vi "Module - RH_RABAR.vi"() -> ()   [LabVIEW 2019]
uses:
  Control/State - eFGV.ctl
panel:
  out "Site Name":string="RH JONATHAN (13.65 kWp)"
  out "STP-03-STATUS":bool
  out "STP-03-B-IDC":dbl caption="B.Idc" format="%.1f A"
  out "STP-03-B-VDC":dbl caption="B.Vdc" format="%.0f V"
  out "STP-03-A-IDC":dbl caption="A.Idc" format="%.1f A"
  out "STP-03-A-VDC":dbl caption="A.Vdc" format="%.0f V"
  out "STP-03-PAC":dbl caption="Pac" format="%#_g W"
  out "BANK-02-TEMP":dbl caption="T_bat" format="%#_g C"
  out "BANK-02-IDC":dbl caption="I_bat" format="%.2f A"
  out "BANK-02-VDC":dbl caption="V_bat" format="%.1f V"
  out "BANK-02-SOC":dbl caption="SOC" format="%#_g %"
  out "PM-01-STATUS":bool
  out "PM-01-FREQ":dbl caption="Freq" format="%.0f Hz"
  out "PM-01-IAC":dbl caption="Iac" format="%.0f A"
  out "PM-01-VAC":dbl caption="Vac" format="%.0f V"
  out "PM-01-PAC":dbl caption="Pac" format="%.0f W"
  out "SI-M-01-STATUS":bool
  out "SI-M-01-FREQ":dbl caption="FREQ" format="%.0f Hz"
  out "SI-M-01-L3":dbl caption="L3" format="%.0f V"
  out "SI-M-01-L2":dbl caption="L2" format="%.0f V"
  out "SI-M-01-L1":dbl caption="L1" format="%.0f V"
  out "SI-M-01-PAC":dbl caption="Pac" format="%.0f W"
  out "BANK-01-TEMP":dbl caption="T_bat" format="%#_g C"
  out "BANK-01-IDC":dbl caption="I_bat" format="%.2f A"
  out "BANK-01-VDC":dbl caption="V_bat" format="%.1f V"
  out "BANK-01-SOC":dbl caption="SOC" format="%#_g %"
  out "STP-02-STATUS":bool
  out "STP-02-B-IDC":dbl caption="B.Idc" format="%.1f A"
  out "STP-02-B-VDC":dbl caption="B.Vdc" format="%.0f V"
  out "STP-02-A-IDC":dbl caption="A.Idc" format="%.1f A"
  out "STP-02-A-VDC":dbl caption="A.Vdc" format="%.0f V"
  out "STP-02-PAC":dbl caption="Pac" format="%#_g W"
  out "STP-01-STATUS":bool
  out "STP-01-B-IDC":dbl caption="B.Idc" format="%.1f A"
  out "STP-01-B-VDC":dbl caption="B.Vdc" format="%.0f V"
  out "STP-01-A-IDC":dbl caption="A.Idc" format="%.1f A"
  out "STP-01-A-VDC":dbl caption="A.Vdc" format="%.0f V"
  out "STP-01-PAC":dbl caption="Pac" format="%.0f W"
  # "RH RABAR (17.29 kWp)"
  # "BANK-1"
  # "BANK-2"
  # "STP-01"
  # "STP-02"
  # "SI-M-01"
  # "STP-03"
  # "PM-01"
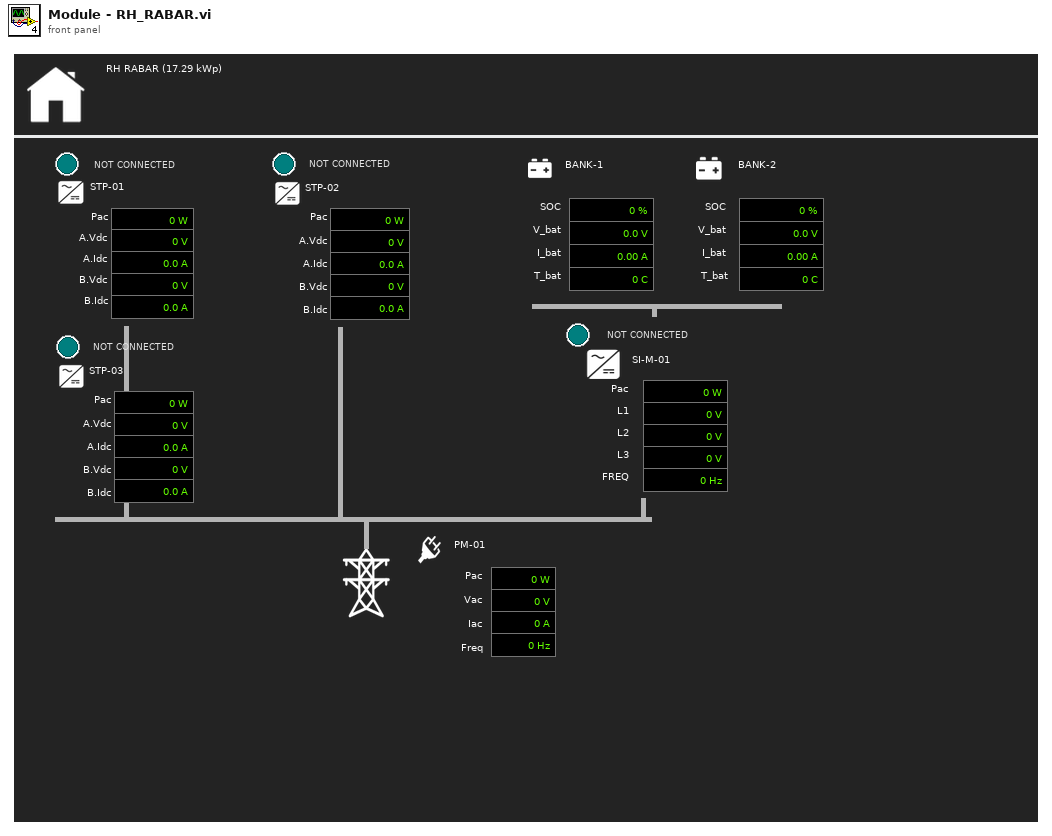
[diagram p1: front panel]
types:
  T1 = typedef "State - eFGV.ctl" = enum16{"Init", "Read", "Write", "Close"}
  T2 = typedef "Device Name.ctl" = enum16{"SB-01", "SB-02", "SB-03", "SB-04", "STP-01", "STP-02", "STP-03", "STP-04", "BANK-01", "BANK-02", "BANK-03", "BANK-04", "SI-M-01", "SI-M-02", "SI-M-03", "SI-M-04", "PM-01", "PM-02", "PM-03", "PM-04"}
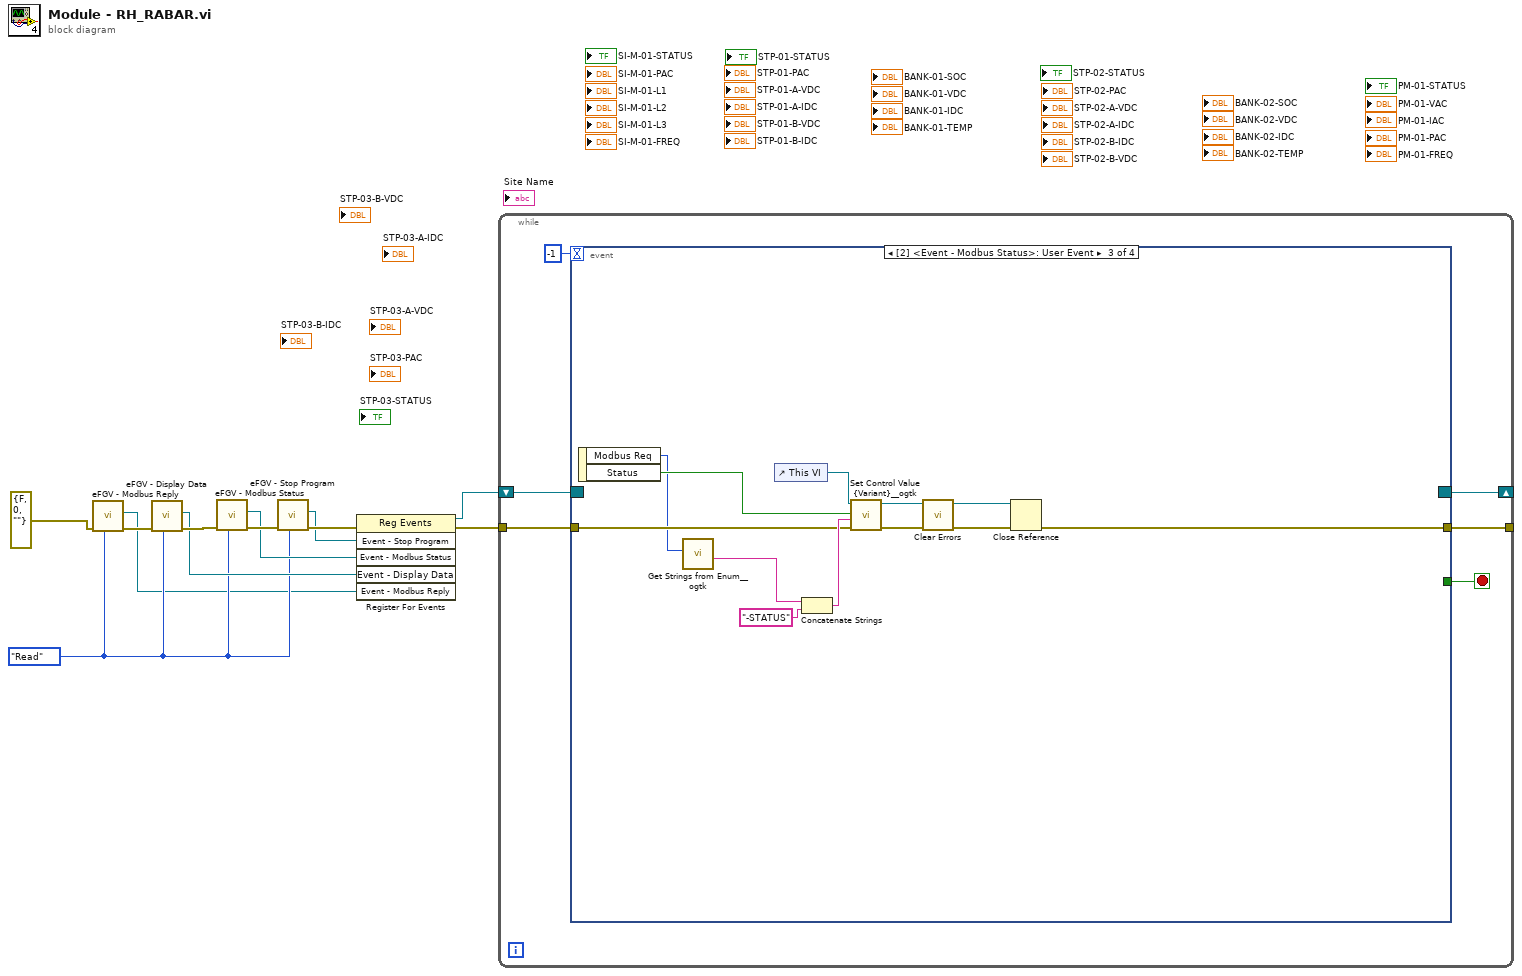
[diagram p0: block diagram]
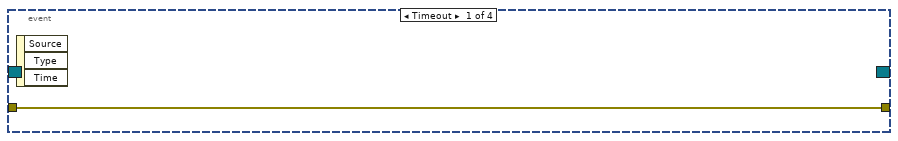
[diagram p2: hidden frame]
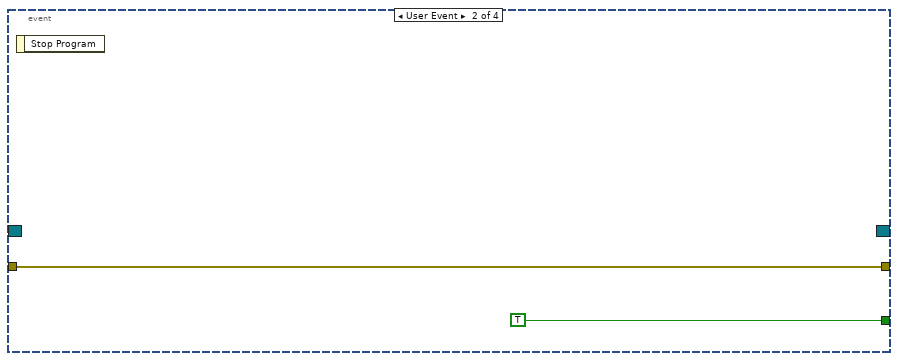
[diagram p3: hidden frame]
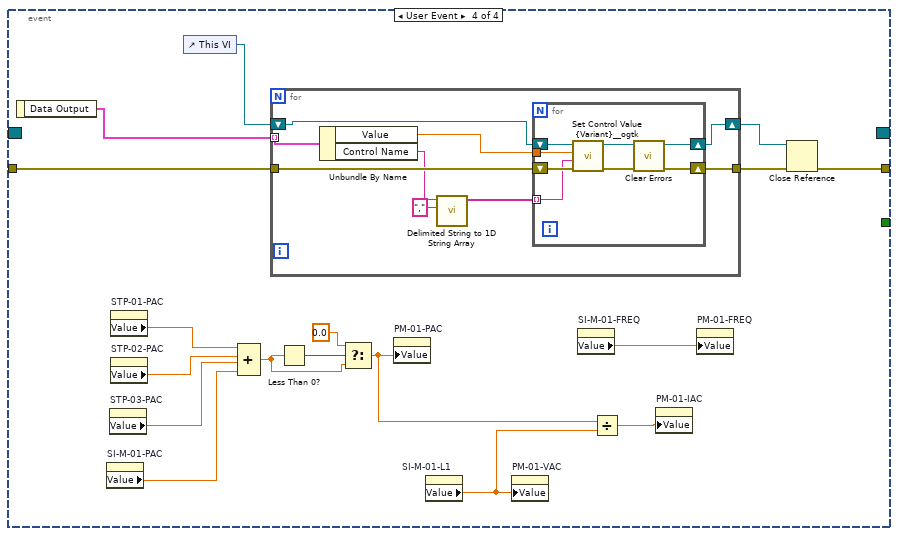
[diagram p4: hidden frame]
diagram:
  w2 = State_-_eFGV."Read" ("State - eFGV")
  n1 = call "eFGV - Modbus Reply.vi"("State - eFGV"=w2, "error in (no error)"=errorcluster {"status"=FALSE, "code"=0, "source"=""}) -> ("error out"=w4:errorcluster, "Event - Modbus Reply"=w1:refnum<user-event>)  [unwired: 8 in]
  n2 = call "eFGV - Display Data.vi"("State - eFGV"=w2, "error in (no error)"=w4) -> ("error out"=w6:errorcluster, "Event - Display Data"=w5:refnum<user-event>)  [unwired: 8 in]
  n3 = call "eFGV - Modbus Status.vi"("State - eFGV"=w2, "error in (no error)"=w6) -> ("error out"=w8:errorcluster, "Event - Modbus Status"=w7:refnum<user-event>)  [unwired: 8 in]
  n4 = call "eFGV - Stop Program.vi"("State - eFGV"=w2, "error in (no error)"=w8) -> ("error out"=w11:errorcluster, "Event - Stop Program"=w10:refnum<user-event>)  [unwired: 8 in]
  n5 = register-events(error in=w11, w10, w7, w5, w1) -> (reference out=w9:refnum<event-registration>, error out=w12:errorcluster)  [unwired: 1 in]
  n6 = while {
    tunnel: w12 -> [w17]
    shift-right: [w16] -> _
    shift-left: w9 -> [w18]
    tunnel: [w13] -> _
    stop <- w15 stop-if-true
    n7 = event shown="[2] <Event - Modbus Status>: User Event" {
      selector: w18 -> [_ _ _ _]
      dyn-events: [_ _ _ _] -> w16
      timeout: -1 -> [_ _ _ _]
      tunnel: w17 -> [w19 w20 w30 w49]
      tunnel: [_ TRUE _ _] -> w15
      tunnel: [w19 w20 w27 w45] -> w13
      event Timeout {
        n8 = event-data() -> ()  [unwired: 1 in, 3 out]
      }
      event User Event {
        n9 = event-data() -> ()  [unwired: 1 in, 1 out]
      }
      event User Event {
        n10 = event-data() -> ("Modbus Req"=w25:T2, "Status"=w29:bool)  [unwired: 1 in]
        n11 = call "Get Strings from Enum__ogtk.vi"("Enum"=w25) -> ("String Value"=w24:string)  [unwired: 7 in, 3 out]
        n12 = control-ref of="This VI"() -> (w32:refnum<vi>)
        n13 = Concatenate Strings(w24, "-STATUS" ("string")) -> (w31:string)
        n14 = call "Set Control Value {Variant}__ogtk.vi"("error in (no error)"=w30, "Control Name (\"\": use variant name)"=w31, "Value"=w29, "VI Refnum"=w32) -> ("error out"=w28:errorcluster, "VI Refnum dup"=w26:refnum<vi>)  [unwired: 6 in]
        n15 = call <vilib>:"Clear Errors.vi"("error in (no error)"=w28) -> ("error out"=w22:errorcluster)  [unwired: 5 in, 1 out]
        n16 = Close Reference(reference=w26, error in (no error)=w22) -> (error out=w27:errorcluster)
      }
      event User Event {
        n17 = event-data() -> ("Data Output"=w46:cluster{"Control Name":string, "Value":dbl}[])  [unwired: 1 in]
        n18 = property on="SI-M-01-PAC" class="DigNum (strict)"() -> ("Value"=w34:dbl)  [unwired: 2 in, 2 out]
        n19 = property on="STP-03-PAC" class="DigNum (strict)"() -> ("Value"=w41:dbl)  [unwired: 2 in, 2 out]
        n20 = property on="STP-01-PAC" class="DigNum (strict)"() -> ("Value"=w43:dbl)  [unwired: 2 in, 2 out]
        n21 = property on="STP-02-PAC" class="DigNum (strict)"() -> ("Value"=w42:dbl)  [unwired: 2 in, 2 out]
        n22 = control-ref of="This VI"() -> (w33:refnum<vi>)
        n23 = Compound Arithmetic op=ADD(w43, w42, w41, w34) -> (w39:dbl)
        n24 = for {
          tunnel: w49 -> [w58]
          tunnel: [w57] -> w48
          tunnel: w46 -> [w55] mode=indexing
          shift-right: [w56] -> w47
          shift-left: w33 -> [w50]
          n25 = Unbundle By Name(w55) -> ("Value"=w54:dbl, "Control Name"=w53:string)
          n26 = call <vilib>:"Delimited String to 1D String Array.vi"("delimiter"=",", "delimited string"=w53) -> ("string array"=w51:string[])  [unwired: 9 in]
          n27 = for {
            tunnel: w54 -> [w61]
            shift-right: [w62] -> w56
            shift-left: w50 -> [w65]
            shift-right: [w59] -> w57
            shift-left: w58 -> [w64]
            tunnel: w51 -> [w60] mode=indexing
            n28 = call "Set Control Value {Variant}__ogtk.vi"("error in (no error)"=w64, "Control Name (\"\": use variant name)"=w60, "Value"=w61, "VI Refnum"=w65) -> ("error out"=w63:errorcluster, "VI Refnum dup"=w62:refnum<vi>)  [unwired: 6 in]
            n29 = call <vilib>:"Clear Errors.vi"("error in (no error)"=w63) -> ("error out"=w59:errorcluster)  [unwired: 5 in, 1 out]
          }
        }
        n30 = Less Than 0?(x=w39) -> (x < 0?=w40:bool)
        n31 = Select(t=0.0, s=w40, f=w39) -> (s? t:f=w36:dbl)
        n32 = property on="PM-01-PAC" class="DigNum (strict)"("Value"=w36) -> ()  [unwired: 2 in, 2 out]
        n33 = property on="SI-M-01-L1" class="DigNum (strict)"() -> ("Value"=w35:dbl)  [unwired: 2 in, 2 out]
        n34 = property on="PM-01-VAC" class="DigNum (strict)"("Value"=w35) -> ()  [unwired: 2 in, 2 out]
        n35 = property on="SI-M-01-FREQ" class="DigNum (strict)"() -> ("Value"=w44:dbl)  [unwired: 2 in, 2 out]
        n36 = Divide(x=w36, y=w35) -> (x/y=w37:dbl)
        n37 = property on="PM-01-IAC" class="DigNum (strict)"("Value"=w37) -> ()  [unwired: 2 in, 2 out]
        n38 = property on="PM-01-FREQ" class="DigNum (strict)"("Value"=w44) -> ()  [unwired: 2 in, 2 out]
        n39 = Close Reference(reference=w47, error in (no error)=w48) -> (error out=w45:errorcluster)
      }
    }
  }
